vi "Init IO Ports.vi"(11 "NotifierReff":T5) -> (1 "Dynamixel Cycles":T1, 2 "Dynamixel Bounds Out":T2, 3 "IO Port Cluster":T4)   [LabVIEW 2013]
doc: "Initializes all I/O ports used and bundles them up for neatness.\n\nEric Schneider, April 2014"
uses:
  Data/TypeDefs/Notifiers.ctl
  Data/TypeDefs/UTM Location.ctl
  Data/TypeDefs/Sail Set Suggestions.ctl
  Data/TypeDefs/Rudder Set Suggestions.ctl
  Data/TypeDefs/OverrideInformation.ctl
  Data/TypeDefs/OverrideMode.ctl
  Data/TypeDefs/MotorSetup.ctl
  Data/TypeDefs/DynamixelSetupInfo.ctl
  Data/TypeDefs/AirmarStatus.ctl
  Data/TypeDefs/HardwareOnline.ctl
  Data/TypeDefs/DynamixelCycleTracker.ctl
  Data/TypeDefs/RC Input Values.ctl
  Classes/Waypoint/Waypoint.lvclass
  Data/TypeDefs/DamnYankeeIOPorts.ctl
  <vilib>/Instr/_visa.llb/VISA Configure Serial Port (Instr).vi
  <vilib>/FPGAPlugInAG/myRIO-1900/niLvFpga_Open_myRIO-1900.vi
  <vilib>/rvi/interface/common/dynamic/niFpgaDynamicAddResources.vi
  <vilib>/rvi/interface/nirviOpenFPGA/nirviOpenFPGA.xnode
  FPGA Bitfiles/AutonomousSailbo_FPGATarget_myRIOPWMDecoder_uSRMj+uIEmA.lvbitx
  FPGA_Code/myRIO_PWM_Decoder.vi
  <instrlib>/Dynamixel Motor/Dynamixel Motor.lvlib
panel:
  out "Motors IDs Found":u8[](array[numeric])
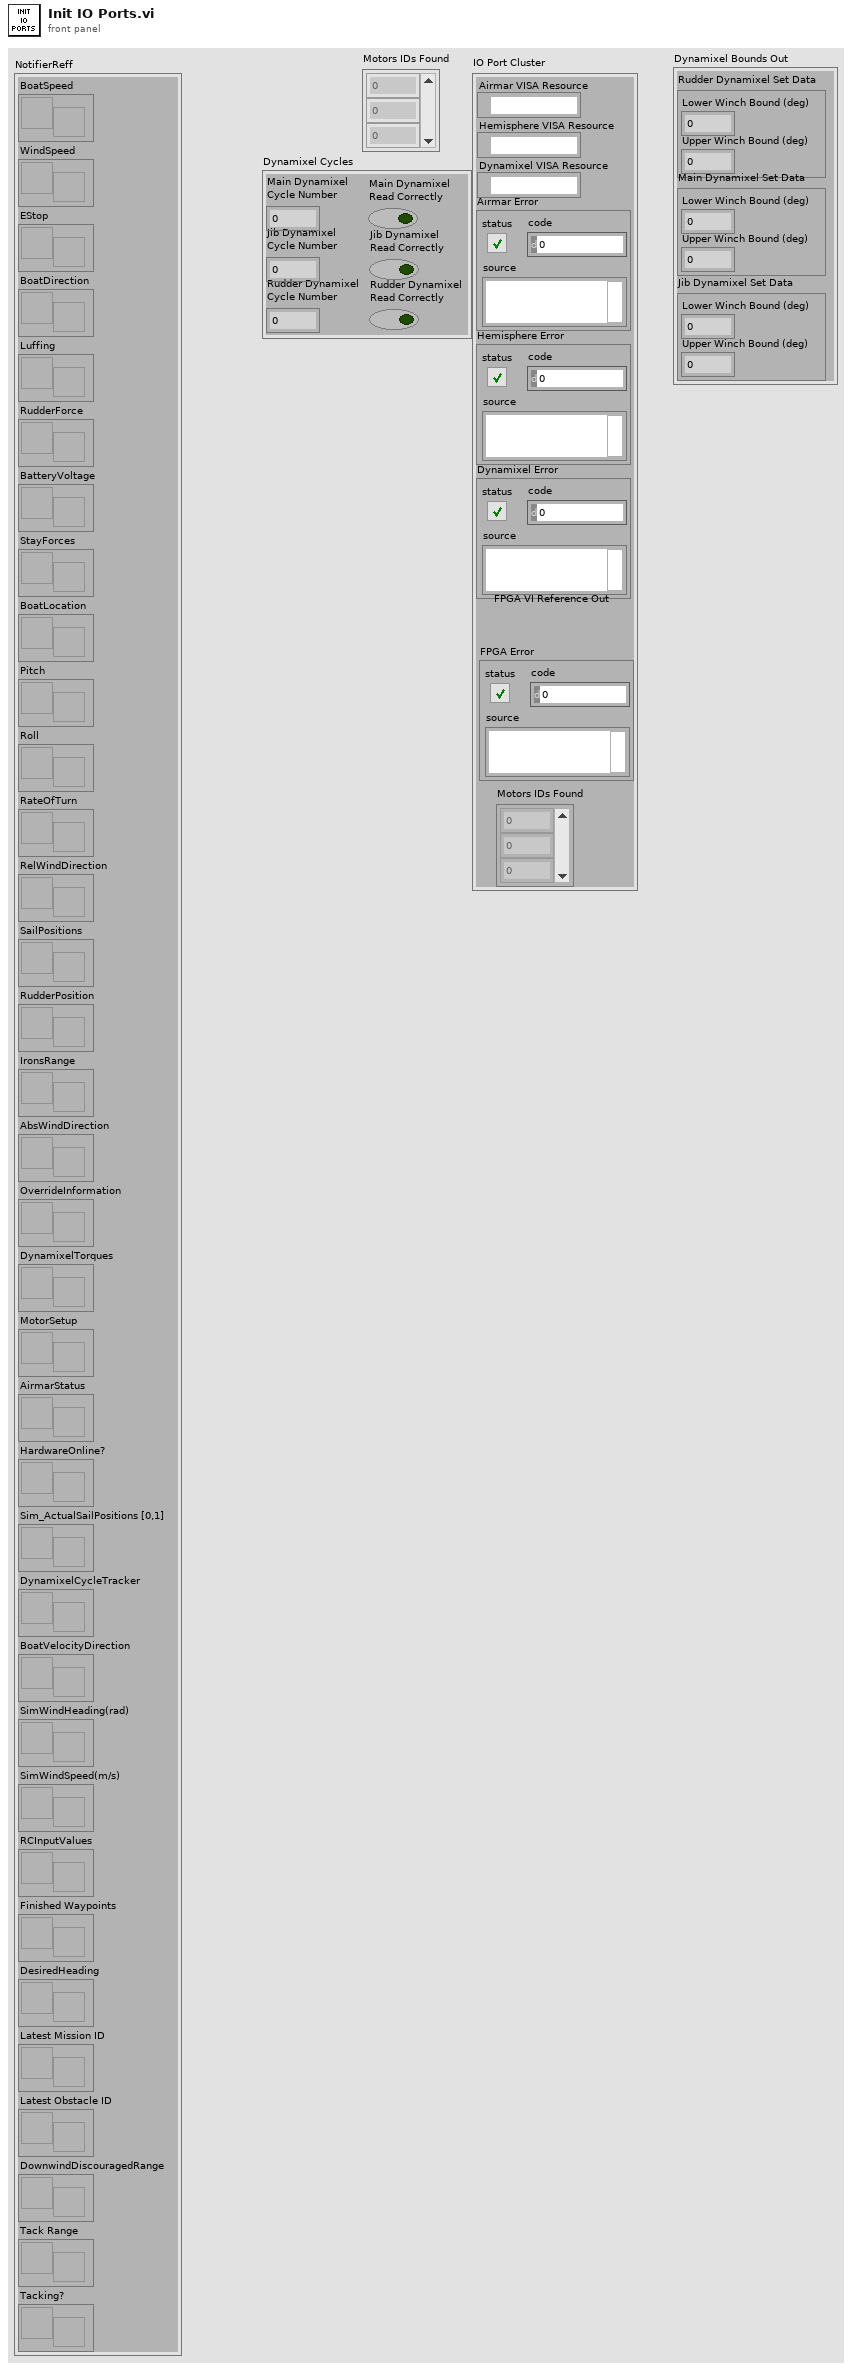
[diagram p1: front panel]
types:
  T1 = typedef "DynamixelCycleTracker.ctl" = cluster{"Main Dynamixel\nCycle Number":i32, "Jib Dynamixel\nCycle Number":i32, "Rudder Dynamixel\nCycle Number":i32, "Main Dynamixel\nRead Correctly":bool, "Jib Dynamixel\nRead Correctly":bool, "Rudder Dynamixel\nRead Correctly":bool}
  T2 = typedef "MotorSetup.ctl" = cluster{"Main Dynamixel Set Data":T3, "Rudder Dynamixel Set Data":T3, "Jib Dynamixel Set Data":T3}
  T3 = typedef "DynamixelSetupInfo.ctl" = cluster{"Lower Winch Bound (deg)":dbl, "Upper Winch Bound (deg)":dbl}
  T4 = typedef "DamnYankeeIOPorts.ctl" = cluster{"Airmar VISA Resource":refnum<visa-resource-name>, "Hemisphere VISA Resource":refnum<visa-resource-name>, "Dynamixel VISA Resource":refnum<visa-resource-name>, "Airmar Error":errorcluster, "Hemisphere Error":errorcluster, "Dynamixel Error":errorcluster, "FPGA Error":errorcluster, "FPGA VI Reference Out":refnum<k20>, "Motors IDs Found":u8[]}
  T5 = typedef "Notifiers.ctl" = cluster{"BoatSpeed":refnum<notifier>, "WindSpeed":refnum<notifier>, "EStop":refnum<notifier>, "BoatDirection":refnum<notifier>, "Luffing":refnum<notifier>, "RudderForce":refnum<notifier>, "BatteryVoltage":refnum<notifier>, "StayForces":refnum<notifier>, "BoatLocation":refnum<notifier>, "Pitch":refnum<notifier>, "Roll":refnum<notifier>, "RateOfTurn":refnum<notifier>, "RelWindDirection":refnum<notifier>, "SailPositions":refnum<notifier>, "RudderPosition":refnum<notifier>, "IronsRange":refnum<notifier>, "AbsWindDirection":refnum<notifier>, "OverrideInformation":refnum<notifier>, "DynamixelTorques":refnum<notifier>, "MotorSetup":refnum<notifier>, "AirmarStatus":refnum<notifier>, "HardwareOnline?":refnum<notifier>, "Sim_ActualSailPositions [0,1]":refnum<notifier>, "DynamixelCycleTracker":refnum<notifier>, "BoatVelocityDirection":refnum<notifier>, "SimWindHeading(rad)":refnum<notifier>, "SimWindSpeed(m/s)":refnum<notifier>, "RCInputValues":refnum<notifier>, "Finished Waypoints":refnum<notifier>, "DesiredHeading":refnum<notifier>, "Latest Mission ID":refnum<notifier>, "Latest Obstacle ID":refnum<notifier>, "DownwindDiscouragedRange":refnum<notifier>, "Tack Range":refnum<notifier>, "Tacking?":refnum<notifier>}
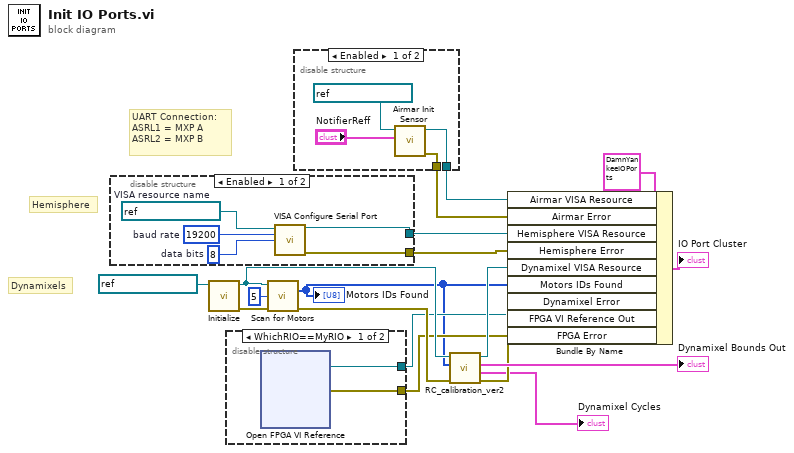
[diagram p0: block diagram]
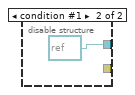
[diagram p4: hidden frame]
diagram:
  # "Dynamixels"
  # "Hemisphere"
  # "UART Connection:\nASRL1 = MXP A \nASRL2 = MXP B"
  n1 = disable-structure shown="Enabled" {
    disable-tunnel: [w23 _] -> w17
    disable-tunnel: [w22 _] -> w16
    frame Enabled {
      w20 = u16 8  # data bits
      w21 = u32 19200  # baud rate
      w19 = refnum<visa-resource-name> "ASRL1::INSTR"  # VISA resource name
      n2 = call-poly "VISA Configure Serial Port"("VISA resource name"=w19, "baud rate (9600)"=w21, "data bits (8)"=w20) -> ("VISA resource name out"=w23:refnum<visa-resource-name>, "error out"=w22:errorcluster)  [unwired: 11 in]
    }
    frame Disabled {
    }
  }
  n3 = call <instrlib>:"Initialize.vi"("VISA resource name"=refnum<visa-resource-name> "ASRL3::INSTR") -> ("error out"=w11:errorcluster, "VISA resource name out"=w9:refnum<visa-resource-name>)  [unwired: 9 in]
  n4 = disable-structure shown="WhichRIO==MyRIO" {
    disable-tunnel: [w25 refnum<k20> refnum ("FPGA VI Reference Out")] -> w3
    disable-tunnel: [w24 _] -> w5
    frame condition #0 (active) {
      n5 = xnode "Open FPGA VI Reference"() -> ("FPGA VI Reference Out"=w25:refnum<k20>, "error out"=w24:errorcluster)  [unwired: 2 in]
    }
    frame condition #1 {
    }
  }
  n6 = call <instrlib>:"Scan for Motors.vi"("VISA resource name"=w9, "Ending ID (253)"=u8 5, "error in (no error)"=w11) -> ("Motors IDs Found"=w2:u8[], "error out"=w8:errorcluster)  [unwired: 10 in, 1 out]
  "Motors IDs Found" <- w2
  n7 = disable-structure shown="Enabled" {
    disable-tunnel: [w30 _] -> w15
    disable-tunnel: [w29 _] -> w14
    frame Enabled {
      n8 = call "Airmar Init Sensor.vi"("NotifierReff"="NotifierReff", "VISA Refnum in"=refnum<visa-resource-name> "ASRL2::INSTR") -> ("error out"=w29:errorcluster, "VISA Refnum out"=w30:refnum<visa-resource-name>)  [unwired: 7 in, 1 out]
    }
    frame Disabled {
    }
  }
  n9 = call "RC_calibration_ver2.vi"("error in (no error)"=w8, "Motors IDs Found"=w2, "VISA resource name"=w9) -> ("error out"=w4:errorcluster, "Dynamixel Cycles"=→"Dynamixel Cycles":T1, "output cluster"=→"Dynamixel Bounds Out":T2, "VISA resource name out"=w7:refnum<visa-resource-name>)  [unwired: 5 in]
  n10 = Bundle By Name(cluster=T4 {"Airmar VISA Resource"="", "Hemisphere VISA Resource"="", "Dynamixel VISA Resource"="", "Airmar Error"={"status"=FALSE, "code"=0, "source"=""}, "Hemisphere Error"={"status"=FALSE, "code"=0, "source"=""}, "Dynamixel Error"={"status"=FALSE, "code"=0, "source"=""}, "FPGA Error"={"status"=FALSE, "code"=0, "source"=""}, "FPGA VI Reference Out"=refnum, "Motors IDs Found"=[]}, "Airmar VISA Resource"=w15, "Airmar Error"=w14, "Hemisphere VISA Resource"=w17, "Hemisphere Error"=w16, "Dynamixel VISA Resource"=w7, "Motors IDs Found"=w2, "Dynamixel Error"=w4, "FPGA VI Reference Out"=w3, "FPGA Error"=w5) -> (→"IO Port Cluster":T4)
